vi "Digital chip test.vi"() -> ()   [LabVIEW 2019]
uses:
  <vilib>/VirtualBench/VirtualBench.lvlib
  <vilib>/Utility/error.llb/DialogType.ctl
  <vilib>/VirtualBench/_PS Configure Voltage Output0.vi
  <vilib>/VirtualBench/_DMM Configure Measurement2.vi
  <vilib>/VirtualBench/_MSO Configure Analog Channel28.vi
  <vilib>/VirtualBench/_FGEN Configure Standard Waveform4.vi
  <vilib>/VirtualBench/_MSO Configure Timing12.vi
  <vilib>/DigilentWF/DigilentWF.lvlib
panel:
  out "VOL(V)":dbl format="%#.2f"
  in  "图表选项卡":enum32{"VOH", "VOL", "电压传输特性"}(tab)
  out "VOH":string[][](table)=[["0", "0", "0", "0"]]
  out "VOL(V)":string[][](table)=[["0", "0", "0", "0"]]
  out "波形图":waveform(dbl)[](graph)
  out "VOH(V)":dbl format="%#.2f"
  out "IIH(μA)":dbl format="%#.2f"
  out "IIL(mA)":dbl format="%#.2f"
  out "ICCH(mA)":dbl format="%#.2f"
  in  "测试参数选项卡":T1(tab)=enum."VOL"
  in  "通道一电压":T2
  in  "测量模式":T3(ring)=enum."DC Current"
  in  "通道一电压 2":T2
  in  "测量模式":T3(ring)=enum."DC Current"
  in  "通道一电压":T2
  in  "测量模式":T3(ring)=enum."DC Current"
  in  "通道一电压 2":T4
  in  "通道一电压":T2
  in  "测量模式":T3(ring)=enum."DC Current"
  in  "通道一电压2":T4
  in  "通道一电压 4":T2
  in  "测量模式":T3(ring)=enum."DC Current"
  in  "通道一电压2 2":T4
  in  "测量模式":T3(ring)=enum."DC Current"
  in  "通道一电压2":T4
  in  "通道一电压":T2
  in  "通道一电压1":T2
  in  "通道一电压2 4":T4
  in  "Amplitude":dbl caption="Amplitude (no change)"
  in  "DC Offset":dbl caption="DC Offset (no change)"
  in  "测量范围":dbl caption="Vertical Range (no change)"
  in  "示波器通道选择":tag caption="Channel"
  in  "Waveform Function":i32(ring) caption="Waveform Function (no change)" items=["Sine", "Square", "Triangle/Ramp", "DC"]
  in  "Frequency":dbl caption="Frequency (no change)"
  out "ICCL(mA)":dbl format="%#.2f"
  in  "测试机台选择":tag="VB8012-3115AD9"
  in  "开始测试":bool caption="Start"
  out "测试进度":u8(slide)=100 caption="Testing..." scale=0.0..100.0
  # "基于IECUBE-3839的74芯片自动化测试程序"
  # "硬件配置"
  # "DUT测试参数"
  # "任务点\n1\n配\n置\n仪\n器\n参\n数"
  # "电源配置"
  # "数字万用表配置"
  # "电源配置"
  # "数字万用表配置"
  # "电源配置"
  # "数字万用表配置"
  # "电源配置"
  # "数字万用表配置"
  # "电源配置"
  # "数字万用表配置"
  # "电源配置"
  # "数字万用表配置"
  # "电源配置"
  # "信号源配置"
  # "示波器配置"
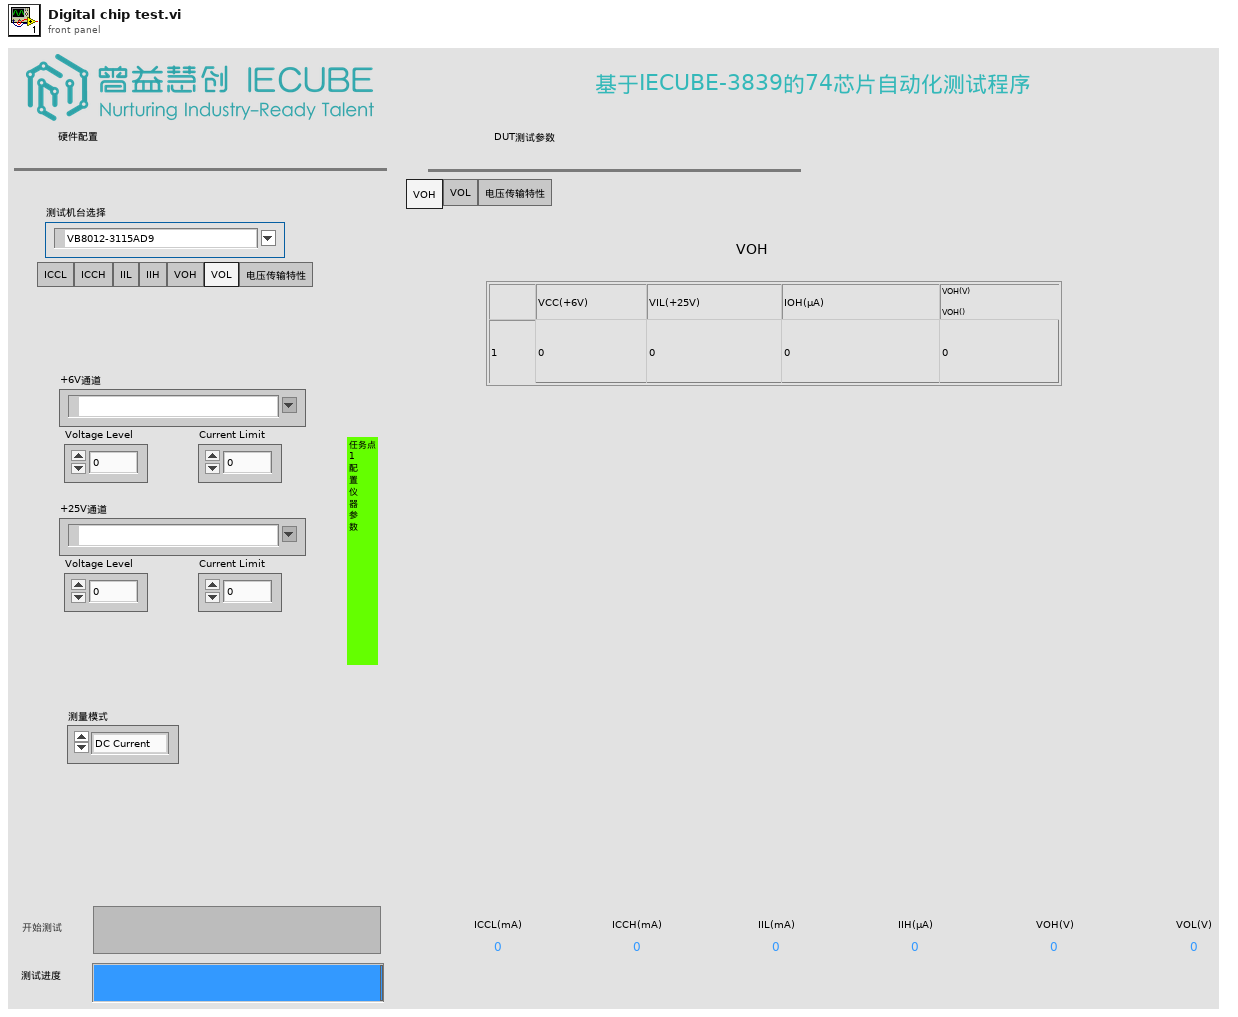
[diagram p1: front panel]
types:
  T1 = enum32{"ICCL", "ICCH", "IIL", "IIH", "VOH", "VOL", "电压传输特性"}
  T2 = cluster{"+6V通道":tag, "Voltage Level":dbl, "Current Limit":dbl}
  T3 = enum16{"DC Volts", "AC Volts", "DC Current", "AC Current", "Resistance", "Diode"}
  T4 = cluster{"+25V通道":tag, "Voltage Level":dbl, "Current Limit":dbl}
  T5 = enum16{"ICCL", "ICCH", "IIL", "IIH", "VOH", "VOL", "电压传输特性"}
  T6 = typedef "DialogType.ctl" = u16
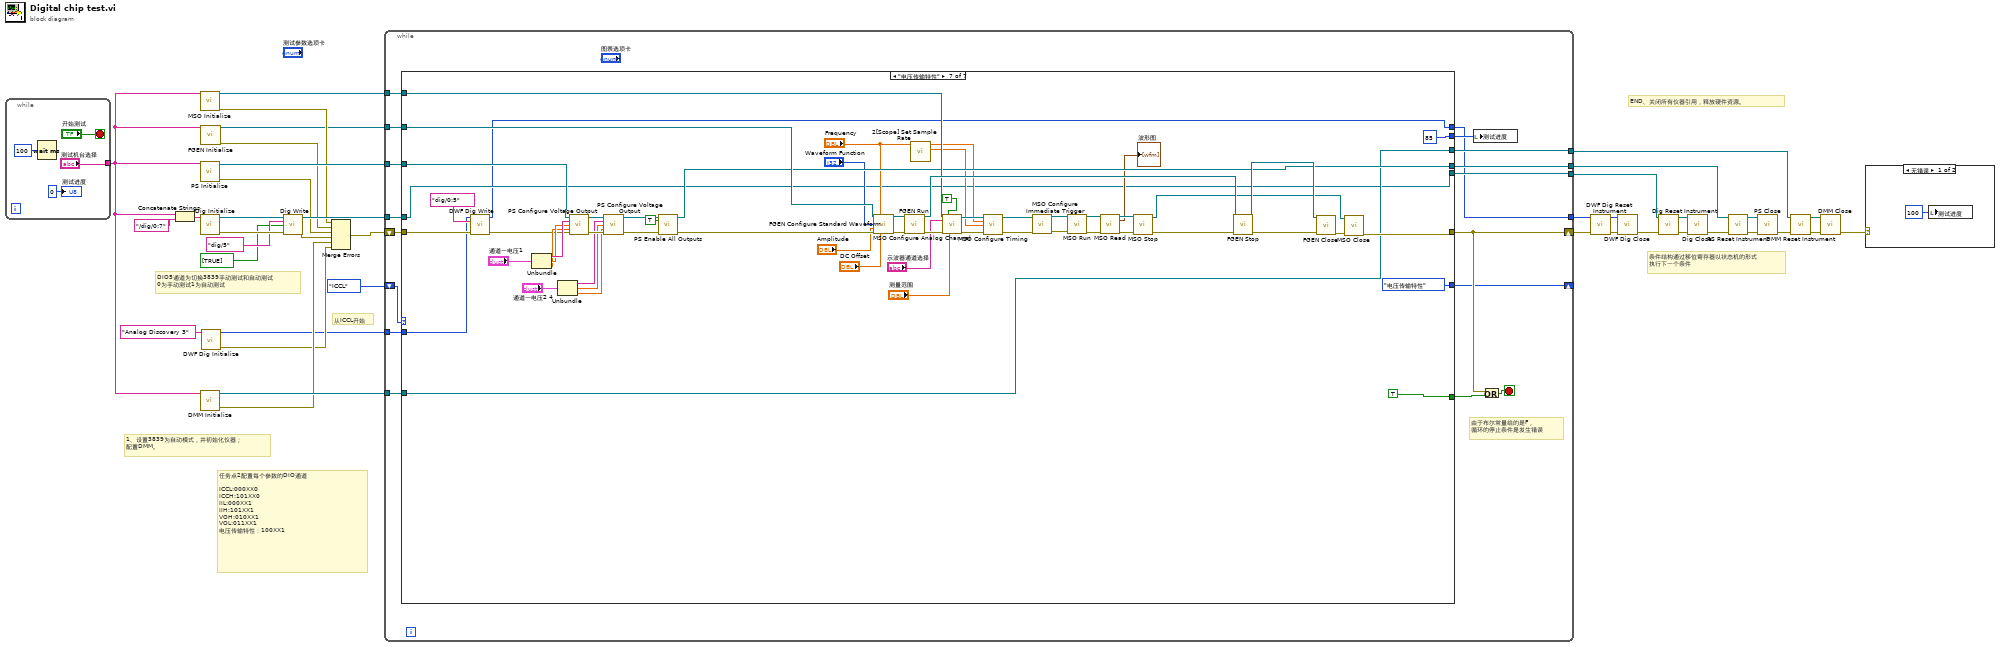
[diagram p0: block diagram]
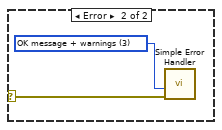
[diagram p2: hidden frame]
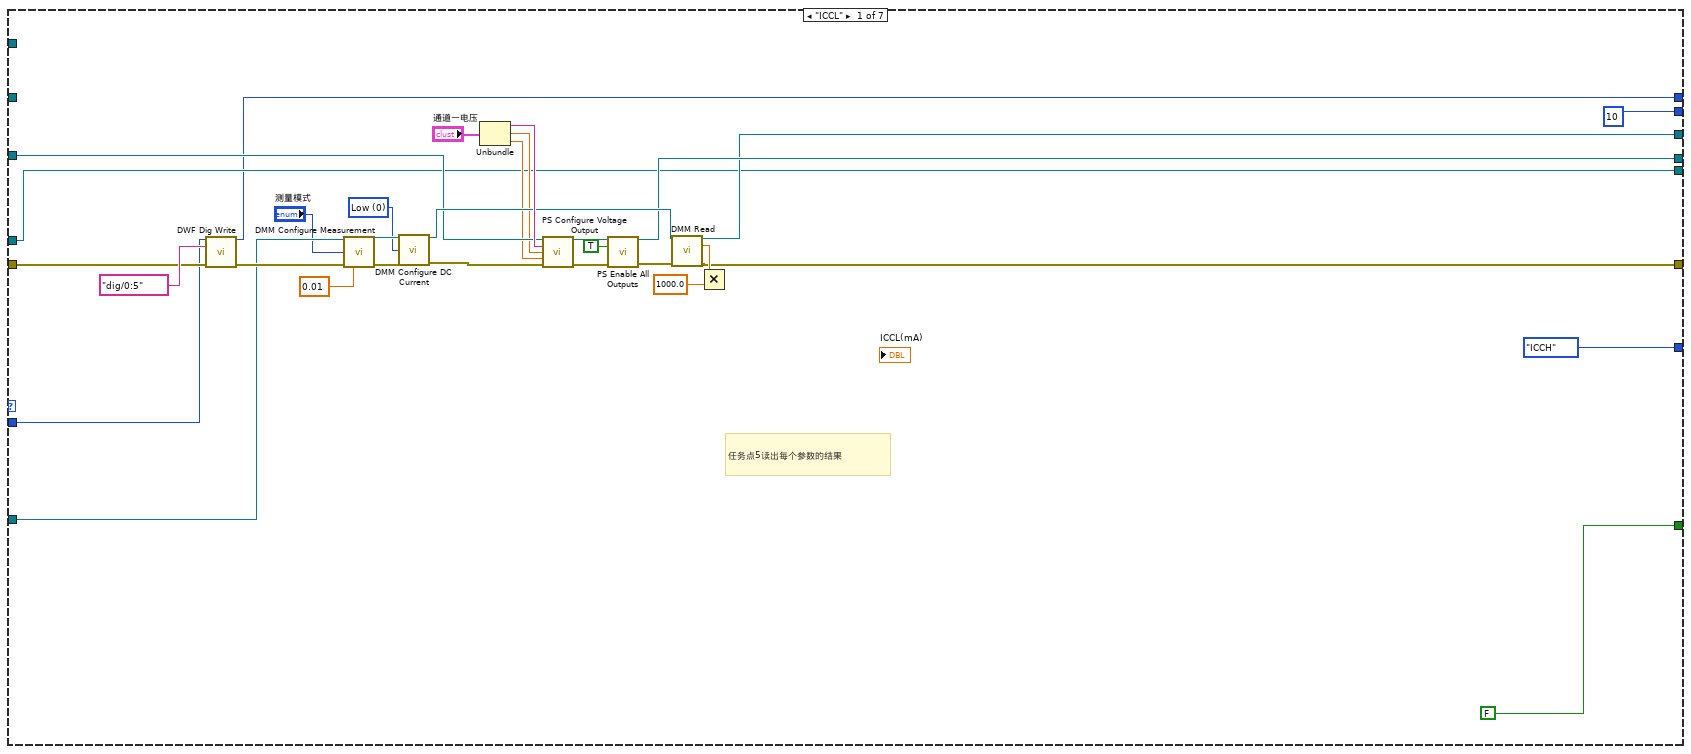
[diagram p3: hidden frame]
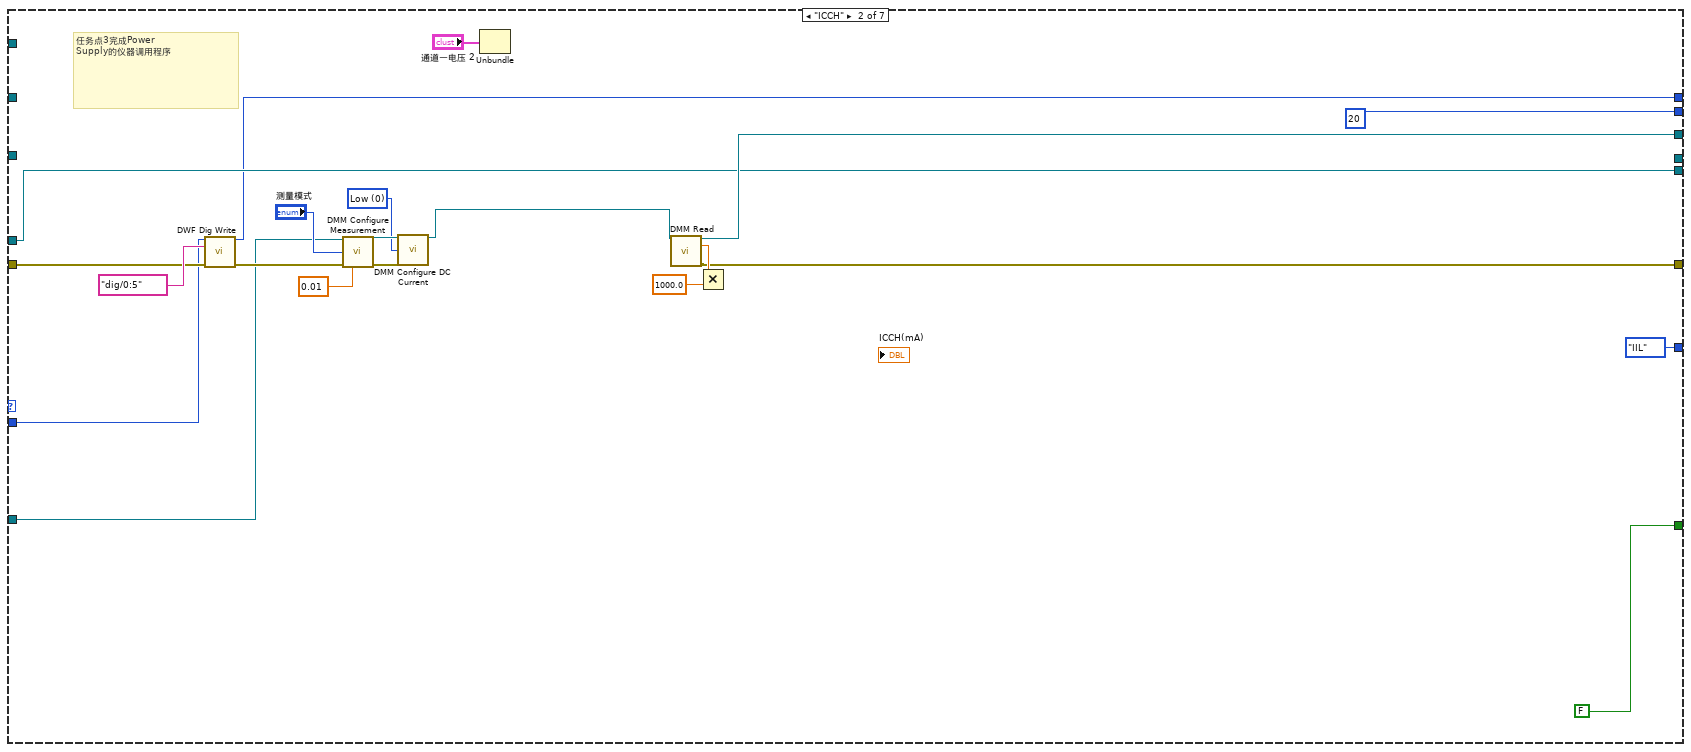
[diagram p4: hidden frame]
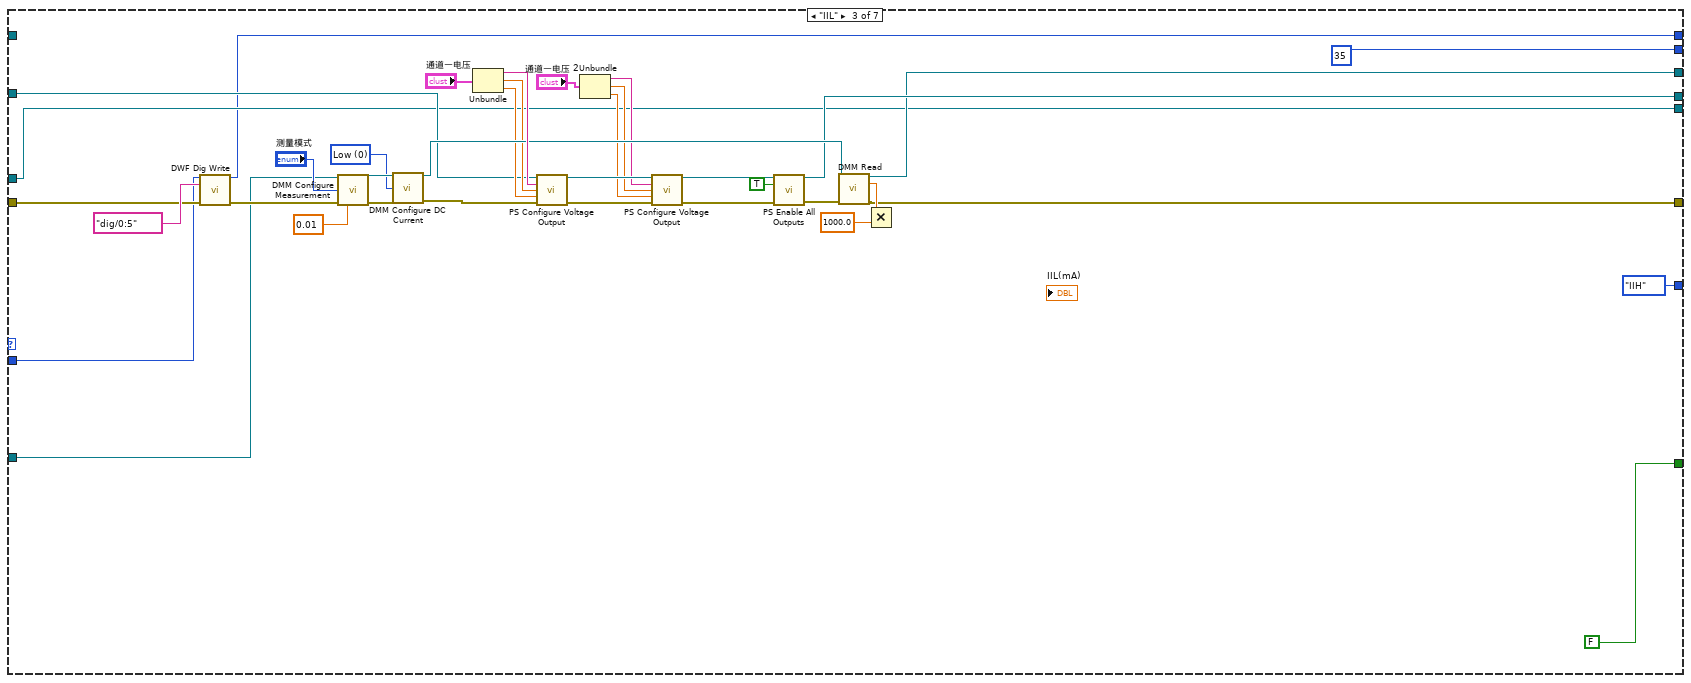
[diagram p5: hidden frame]
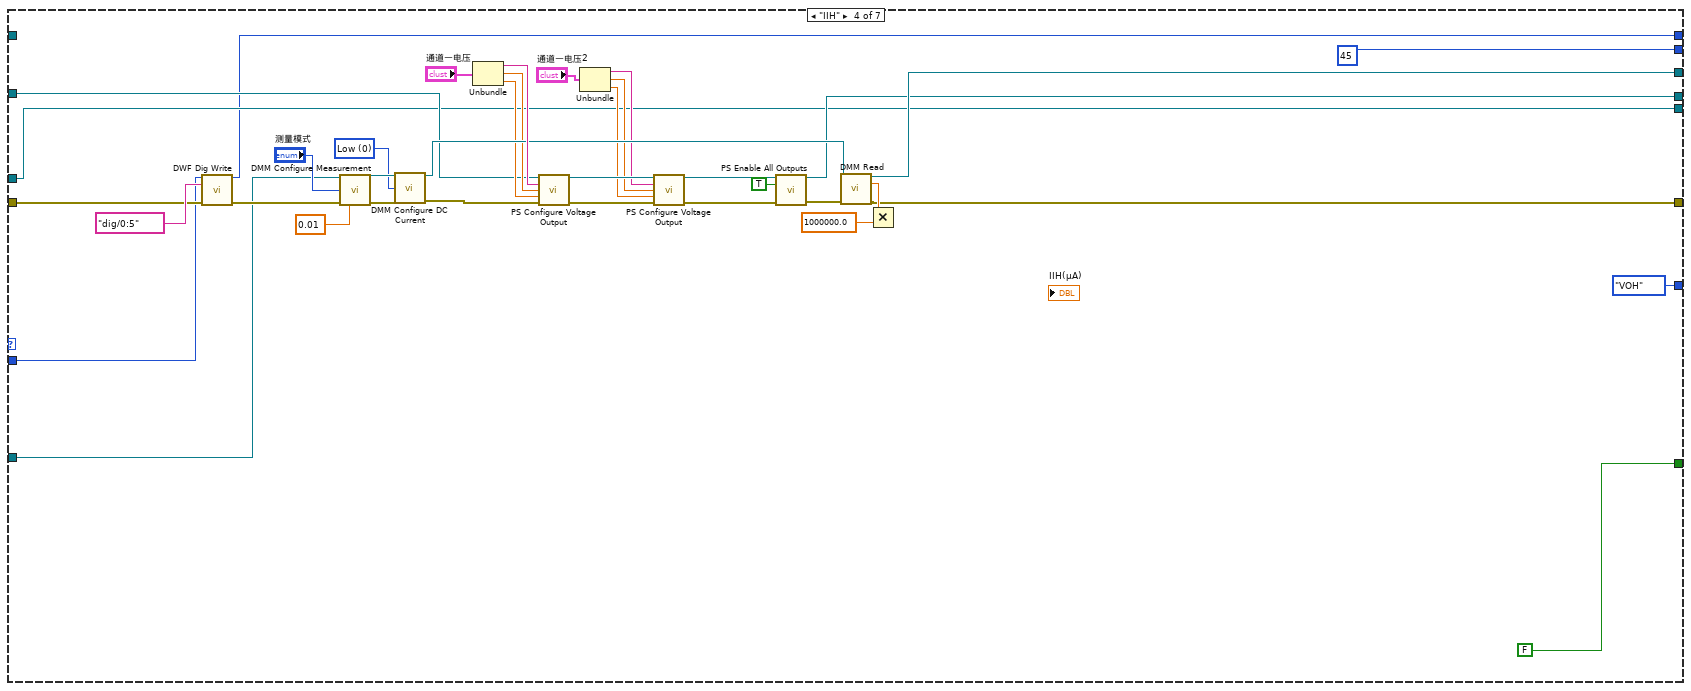
[diagram p6: hidden frame]
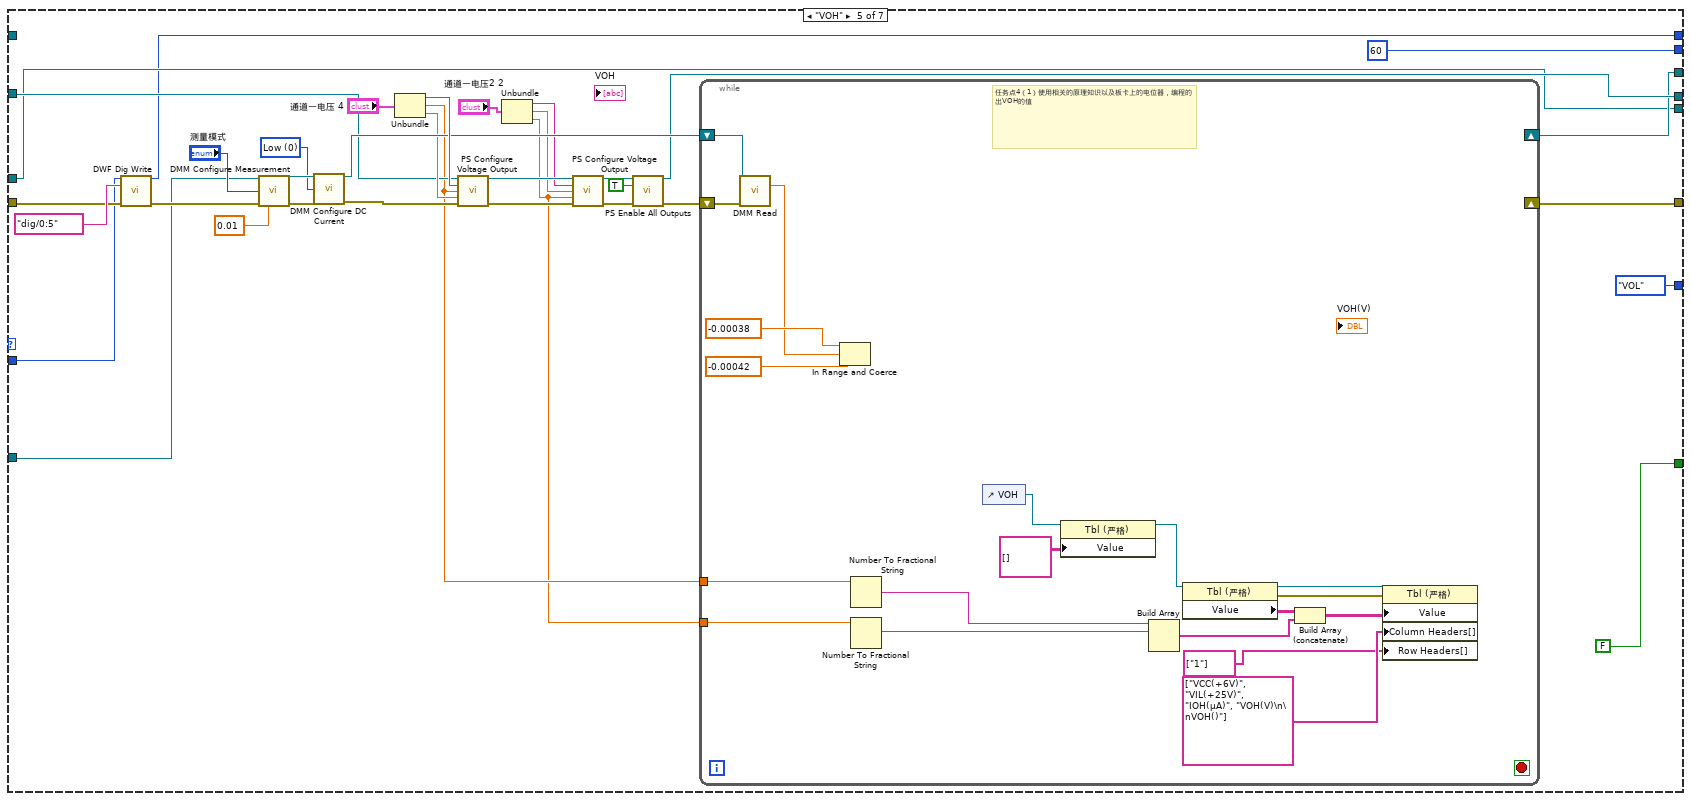
[diagram p7: hidden frame]
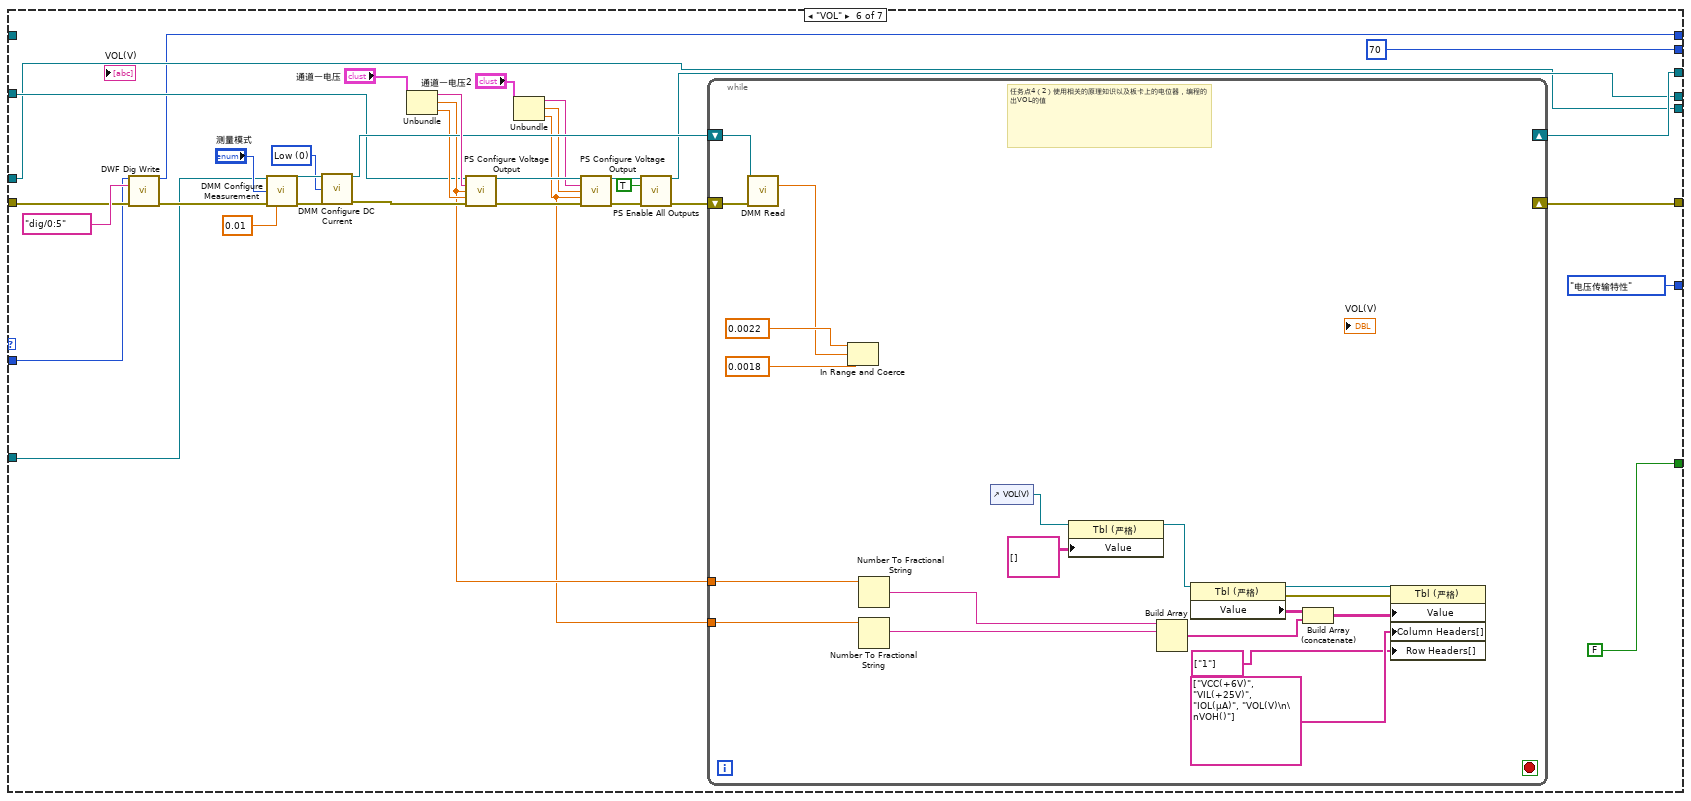
[diagram p8: hidden frame]
diagram:
  # "任务点2配置每个参数的DIO通道\n\nICCL:000XX0\nICCH:101XX0\nIIL:000XX1\nIIH:101XX1\nVOH:010XX1\nVOL:011XX1\n电压传输特性：100XX1"
  # "条件结构通过移位寄存器以状态机的形式\n执行下一个条件"
  # "从ICCL开始"
  # "DIO5通道为切换3839手动测试和自动测试\n0为手动测试1为自动测试"
  # "END、关闭所有仪器引用，释放硬件资源。"
  # "1、设置3839为自动模式，并初始化仪器；\n配置DMM。"
  n1 = while {
    tunnel: ["测试机台选择"] -> w14
    stop <- "开始测试" stop-if-true
    n2 = Wait (ms)(milliseconds to wait=u32 100 ("等待时间（毫秒）")) -> ()  [unwired: 1 out]
    "测试进度" <- u8 0 ("测试进度")
  }
  n3 = Concatenate Strings(w14, "/dig/0:7" ("字符串")) -> (w34:string)
  n4 = call <vilib>:"MSO Initialize.vi"("Device Name"=w14) -> ("Instrument Handle Out"=w11:refnum<k21>, "Error Out"=w12:errorcluster)  [unwired: 13 in]
  n5 = call <vilib>:"PS Initialize.vi"("Device Name"=w14) -> ("Instrument Handle Out"=w33:refnum<k21>, "Error Out"=w30:errorcluster)  [unwired: 13 in]
  n6 = call <vilib>:"Dig Initialize.vi"("Lines"=w34) -> ("Instrument Handle Out"=w39:refnum<k21>, "Error Out"=w38:errorcluster)  [unwired: 13 in]
  n7 = call <vilib>:"DMM Initialize.vi"("Device Name"=w14) -> ("Instrument Handle Out"=w28:refnum<k21>, "Error Out"=w27:errorcluster)  [unwired: 13 in]
  n8 = call <vilib>:"FGEN Initialize.vi"("Device Name"=w14) -> ("Instrument Handle Out"=w10:refnum<k21>, "Error Out"=w13:errorcluster)  [unwired: 13 in]
  n9 = call <vilib>:"DWF Dig Initialize.vi"("Device Name/Lines"="Analog Discovery 3") -> ("Instrument Handle Out"=w6:u32, "Error Out"=w7:errorcluster)  [unwired: 13 in]
  n10 = call <vilib>:"Dig Write.vi"("Instrument Handle In"=w39, "Lines"=tag "dig/5", "Data"=bool[] [TRUE], "Error In"=w38) -> ("Instrument Handle Out"=w32:refnum<k21>, "Error Out"=w29:errorcluster)  [unwired: 10 in]
  n11 = Merge Errors(w12, w13, w30, w29, w27, w7) -> (w31:errorcluster)
  n12 = while {
    tunnel: w32 -> [w44]
    tunnel: w33 -> [w58]
    tunnel: w28 -> [w60]
    shift-right: [w52] -> w5
    shift-left: w31 -> [w59]
    tunnel: [w51] -> w17
    tunnel: [w57] -> w23
    tunnel: [w53] -> w15
    tunnel: w11 -> [w50]
    tunnel: w10 -> [w49]
    shift-right: [w47] -> _
    shift-left: T5."ICCL" -> [w48]
    tunnel: w6 -> [w46]
    tunnel: [w45] -> w1
    stop <- w54 stop-if-true
    # "由于布尔常量给的是F，\n循环的停止条件是发生错误"
    n13 = case shown="\"电压传输特性\"" w48 {
      tunnel: w60 -> [w75 w100 w132 w161 w200 w262 w329]
      tunnel: w59 -> [w77 w101 w133 w162 w201 w263 w340]
      tunnel: w44 -> [w63 w94 w117 w154 w191 w253 w316]
      tunnel: w58 -> [w73 _ w134 w163 w202 w264 w338]
      tunnel: [w65 w99 w129 w159 w197 w260 w329] -> w51
      tunnel: [w72 _ w130 w158 w198 w259 w332] -> w57
      tunnel: [u8 10 ("测试进度") u8 20 ("测试进度") u8 35 ("测试进度") u8 45 ("测试进度") u8 60 ("测试进度") u8 70 ("测试进度") u8 85 ("测试进度")] -> w56
      tunnel: [FALSE FALSE FALSE FALSE FALSE FALSE TRUE] -> w55
      tunnel: [w63 w94 w117 w154 w191 w253 w316] -> w53
      tunnel: [w66 w97 w131 w157 w199 w261 w330] -> w52
      tunnel: w50 -> [_ _ _ _ _ _ w335]
      tunnel: w49 -> [_ _ _ _ _ _ w334]
      tunnel: [T5."ICCH" T5."IIL" T5."IIH" T5."VOH" T5."VOL" T5."电压传输特性" T5."电压传输特性"] -> w47
      tunnel: w46 -> [w61 w92 w116 w153 w190 w252 w315]
      tunnel: [w62 w93 w115 w152 w189 w251 w314] -> w45
      frame "ICCL" {
        w88 = 0 items=["Low", "High"] ("Auto Range Terminal")
        # "任务点5读出每个参数的结果"
        n14 = call <vilib>:"DWF Dig Write.vi"("Instrument Handle In"=w61, "Lines"=tag "dig/0:5", "Error In"=w77) -> ("Instrument Handle Out"=w62:u32, "Error Out"=w76:errorcluster)  [unwired: 11 in]
        n15 = call-poly <vilib>:"DMM Configure Measurement.vi"("Instrument Handle In"=w75, "Function"="测量模式", "Error In"=w76, "Manual Range"=0.01) -> ("Instrument Handle Out"=w89:refnum<k21>, "Error Out"=w90:errorcluster)  [unwired: 10 in]
        n16 = call <vilib>:"DMM Configure DC Current.vi"("Instrument Handle In"=w89, "Auto Range Terminal"=w88, "Error In"=w90) -> ("Instrument Handle Out"=w81:refnum<k21>, "Error Out"=w74:errorcluster)  [unwired: 11 in]
        n17 = Unbundle("通道一电压") -> ("+6V通道"=w85:tag, "Voltage Level"=w68:dbl, "Current Limit"=w69:dbl)
        n18 = call-poly <vilib>:"PS Configure Voltage Output.vi"("Instrument Handle In"=w73, "Channel"=w85, "Voltage Level"=w68, "Current Limit"=w69, "Error In"=w74) -> ("Instrument Handle Out"=w84:refnum<k21>, "Error Out"=w83:errorcluster)  [unwired: 9 in]
        n19 = call <vilib>:"PS Enable All Outputs.vi"("Instrument Handle In"=w84, "Enable Outputs"=TRUE, "Error In"=w83) -> ("Instrument Handle Out"=w72:refnum<k21>, "Error Out"=w80:errorcluster)  [unwired: 11 in]
        n20 = call <vilib>:"DMM Read.vi"("Instrument Handle In"=w81, "Error In"=w80) -> ("Instrument Handle Out"=w65:refnum<k21>, "Measurement"=w79:dbl, "Error Out"=w66:errorcluster)  [unwired: 11 in]
        n21 = Multiply(x=w79, y=1000.0) -> ()  [unwired: 1 out]
      }
      frame "ICCH" {
        w112 = 0 items=["Low", "High"] ("Auto Range Terminal")
        # "任务点3完成Power Supply的仪器调用程序"
        n22 = call <vilib>:"DWF Dig Write.vi"("Instrument Handle In"=w92, "Lines"=tag "dig/0:5", "Error In"=w101) -> ("Instrument Handle Out"=w93:u32, "Error Out"=w105:errorcluster)  [unwired: 11 in]
        n23 = call-poly <vilib>:"DMM Configure Measurement.vi"("Instrument Handle In"=w100, "Function"="测量模式", "Error In"=w105, "Manual Range"=0.01) -> ("Instrument Handle Out"=w113:refnum<k21>, "Error Out"=w114:errorcluster)  [unwired: 10 in]
        n24 = call <vilib>:"DMM Configure DC Current.vi"("Instrument Handle In"=w113, "Auto Range Terminal"=w112, "Error In"=w114) -> ("Instrument Handle Out"=w109:refnum<k21>, "Error Out"=w104:errorcluster)  [unwired: 11 in]
        n25 = Unbundle("通道一电压 2") -> ()  [unwired: 3 out]
        n26 = call <vilib>:"DMM Read.vi"("Instrument Handle In"=w109) -> ("Instrument Handle Out"=w99:refnum<k21>, "Measurement"=w107:dbl, "Error In"=w108:errorcluster, "Error Out"=w97:errorcluster)  [unwired: 11 in]
        n27 = Multiply(x=w107, y=1000.0) -> ()  [unwired: 1 out]
      }
      frame "IIL" {
        w149 = 0 items=["Low", "High"] ("Auto Range Terminal")
        n28 = call <vilib>:"DWF Dig Write.vi"("Instrument Handle In"=w116, "Lines"=tag "dig/0:5", "Error In"=w133) -> ("Instrument Handle Out"=w115:u32, "Error Out"=w140:errorcluster)  [unwired: 11 in]
        n29 = call-poly <vilib>:"DMM Configure Measurement.vi"("Instrument Handle In"=w132, "Function"="测量模式", "Error In"=w140, "Manual Range"=0.01) -> ("Instrument Handle Out"=w150:refnum<k21>, "Error Out"=w151:errorcluster)  [unwired: 10 in]
        n30 = call <vilib>:"DMM Configure DC Current.vi"("Instrument Handle In"=w150, "Auto Range Terminal"=w149, "Error In"=w151) -> ("Instrument Handle Out"=w144:refnum<k21>, "Error Out"=w139:errorcluster)  [unwired: 11 in]
        n31 = Unbundle("通道一电压") -> ("+6V通道"=w146:tag, "Voltage Level"=w136:dbl, "Current Limit"=w137:dbl)
        n32 = call-poly <vilib>:"PS Configure Voltage Output.vi"("Instrument Handle In"=w134, "Channel"=w146, "Voltage Level"=w136, "Current Limit"=w137, "Error In"=w139) -> ("Instrument Handle Out"=w126:refnum<k21>, "Error Out"=w123:errorcluster)  [unwired: 9 in]
        n33 = Unbundle("通道一电压 2") -> ("+25V通道"=w122:tag, "Voltage Level"=w121:dbl, "Current Limit"=w120:dbl)
        n34 = call-poly <vilib>:"PS Configure Voltage Output.vi"("Instrument Handle In"=w126, "Channel"=w122, "Voltage Level"=w121, "Current Limit"=w120, "Error In"=w123) -> ("Instrument Handle Out"=w125:refnum<k21>, "Error Out"=w124:errorcluster)  [unwired: 9 in]
        n35 = call <vilib>:"PS Enable All Outputs.vi"("Instrument Handle In"=w125, "Enable Outputs"=TRUE, "Error In"=w124) -> ("Instrument Handle Out"=w130:refnum<k21>, "Error Out"=w143:errorcluster)  [unwired: 11 in]
        n36 = call <vilib>:"DMM Read.vi"("Instrument Handle In"=w144, "Error In"=w143) -> ("Instrument Handle Out"=w129:refnum<k21>, "Measurement"=w142:dbl, "Error Out"=w131:errorcluster)  [unwired: 11 in]
        n37 = Multiply(x=w142, y=1000.0) -> ()  [unwired: 1 out]
      }
      frame "IIH" {
        w186 = 0 items=["Low", "High"] ("Auto Range Terminal")
        n38 = call <vilib>:"DWF Dig Write.vi"("Instrument Handle In"=w153, "Lines"=tag "dig/0:5", "Error In"=w162) -> ("Instrument Handle Out"=w152:u32, "Error Out"=w177:errorcluster)  [unwired: 11 in]
        n39 = call-poly <vilib>:"DMM Configure Measurement.vi"("Instrument Handle In"=w161, "Function"="测量模式", "Error In"=w177, "Manual Range"=0.01) -> ("Instrument Handle Out"=w187:refnum<k21>, "Error Out"=w188:errorcluster)  [unwired: 10 in]
        n40 = call <vilib>:"DMM Configure DC Current.vi"("Instrument Handle In"=w187, "Auto Range Terminal"=w186, "Error In"=w188) -> ("Instrument Handle Out"=w181:refnum<k21>, "Error Out"=w176:errorcluster)  [unwired: 11 in]
        n41 = Unbundle("通道一电压") -> ("+6V通道"=w183:tag, "Voltage Level"=w173:dbl, "Current Limit"=w174:dbl)
        n42 = call-poly <vilib>:"PS Configure Voltage Output.vi"("Instrument Handle In"=w163, "Channel"=w183, "Voltage Level"=w173, "Current Limit"=w174, "Error In"=w176) -> ("Instrument Handle Out"=w170:refnum<k21>, "Error Out"=w167:errorcluster)  [unwired: 9 in]
        n43 = Unbundle("通道一电压2") -> ("+25V通道"=w166:tag, "Voltage Level"=w165:dbl, "Current Limit"=w164:dbl)
        n44 = call-poly <vilib>:"PS Configure Voltage Output.vi"("Instrument Handle In"=w170, "Channel"=w166, "Voltage Level"=w165, "Current Limit"=w164, "Error In"=w167) -> ("Instrument Handle Out"=w169:refnum<k21>, "Error Out"=w168:errorcluster)  [unwired: 9 in]
        n45 = call <vilib>:"PS Enable All Outputs.vi"("Instrument Handle In"=w169, "Enable Outputs"=TRUE, "Error In"=w168) -> ("Instrument Handle Out"=w158:refnum<k21>, "Error Out"=w180:errorcluster)  [unwired: 11 in]
        n46 = call <vilib>:"DMM Read.vi"("Instrument Handle In"=w181, "Error In"=w180) -> ("Instrument Handle Out"=w159:refnum<k21>, "Measurement"=w179:dbl, "Error Out"=w157:errorcluster)  [unwired: 11 in]
        n47 = Multiply(x=w179, y=1000000.0) -> ()  [unwired: 1 out]
      }
      frame "VOH" {
        w221 = 0 items=["Low", "High"] ("Auto Range Terminal")
        n48 = call <vilib>:"DWF Dig Write.vi"("Instrument Handle In"=w190, "Lines"=tag "dig/0:5", "Error In"=w201) -> ("Instrument Handle Out"=w189:u32, "Error Out"=w214:errorcluster)  [unwired: 11 in]
        n49 = call-poly <vilib>:"DMM Configure Measurement.vi"("Instrument Handle In"=w200, "Function"="测量模式", "Error In"=w214, "Manual Range"=0.01) -> ("Instrument Handle Out"=w222:refnum<k21>, "Error Out"=w223:errorcluster)  [unwired: 10 in]
        n50 = call <vilib>:"DMM Configure DC Current.vi"("Instrument Handle In"=w222, "Auto Range Terminal"=w221, "Error In"=w223) -> ("Instrument Handle Out"=w216:refnum<k21>, "Error Out"=w213:errorcluster)  [unwired: 11 in]
        n51 = Unbundle("通道一电压 4") -> ("+6V通道"=w218:tag, "Voltage Level"=w195:dbl, "Current Limit"=w211:dbl)
        n52 = call-poly <vilib>:"PS Configure Voltage Output.vi"("Instrument Handle In"=w202, "Channel"=w218, "Voltage Level"=w195, "Current Limit"=w211, "Error In"=w213) -> ("Instrument Handle Out"=w208:refnum<k21>, "Error Out"=w205:errorcluster)  [unwired: 9 in]
        n53 = Unbundle("通道一电压2 2") -> ("+25V通道"=w204:tag, "Voltage Level"=w203:dbl, "Current Limit"=w194:dbl)
        n54 = call-poly <vilib>:"PS Configure Voltage Output.vi"("Instrument Handle In"=w208, "Channel"=w204, "Voltage Level"=w203, "Current Limit"=w194, "Error In"=w205) -> ("Instrument Handle Out"=w207:refnum<k21>, "Error Out"=w206:errorcluster)  [unwired: 9 in]
        n55 = call <vilib>:"PS Enable All Outputs.vi"("Instrument Handle In"=w207, "Enable Outputs"=TRUE, "Error In"=w206) -> ("Instrument Handle Out"=w198:refnum<k21>, "Error Out"=w215:errorcluster)  [unwired: 11 in]
        n56 = while {
          shift-right: [w243] -> w197
          shift-left: w216 -> [w250]
          shift-right: [w242] -> w199
          shift-left: w215 -> [w249]
          tunnel: w195 -> [w226]
          tunnel: w194 -> [w225]
          stop <- w224 stop-if-true
          # "任务点4（1）使用相关的原理知识以及板卡上的电位器，编程的出VOH的值"
          n57 = call <vilib>:"DMM Read.vi"("Instrument Handle In"=w250, "Error In"=w249) -> ("Instrument Handle Out"=w245:refnum<k21>, "Measurement"=w241:dbl, "Error Out"=w244:errorcluster)  [unwired: 11 in]
          n58 = In Range and Coerce(upper limit=-0.00038 ("上限"), x=w241, lower limit=-0.00042 ("下限")) -> (In Range?=w246:bool)  [unwired: 1 out]
          n59 = Number To Fractional String(number=w226) -> (F-format string=w240:string)  [unwired: 3 in]
          n60 = Number To Fractional String(number=w225) -> (F-format string=w233:string)  [unwired: 3 in]
          n61 = control-ref of="VOH"() -> (w229:refnum<vi>)
          n62 = property class="Tbl (严格)"(reference=w229, "Value"=string[][] [] ("值")) -> (reference out=w235:refnum<vi>)  [unwired: 1 in, 1 out]
          n63 = Build Array(w240, w233) -> (w234:string[], w227:string, w228:string)
          n64 = property class="Tbl (严格)"(reference=w235) -> (reference out=w238:refnum<vi>, error out=w239:errorcluster, "Value"=w237:string[][])  [unwired: 1 in]
          n65 = Build Array (concatenate)(w237, w234) -> (w236:string[][])
          n66 = property class="Tbl (严格)"(reference=w238, error in=w239, "Value"=w236, "Column Headers[]"=string[] ["VCC(+6V)", "VIL(+25V)", "IOH(μA)", "VOH(V)\n\nVOH()"] ("列首字符串[]"), "Row Headers[]"=string[] ["1"] ("列首字符串[]")) -> ()  [unwired: 2 out]
        }
      }
      frame "VOL" {
        w283 = 0 items=["Low", "High"] ("Auto Range Terminal")
        n67 = call <vilib>:"DWF Dig Write.vi"("Instrument Handle In"=w252, "Lines"=tag "dig/0:5", "Error In"=w263) -> ("Instrument Handle Out"=w251:u32, "Error Out"=w276:errorcluster)  [unwired: 11 in]
        n68 = call-poly <vilib>:"DMM Configure Measurement.vi"("Instrument Handle In"=w262, "Function"="测量模式", "Error In"=w276, "Manual Range"=0.01) -> ("Instrument Handle Out"=w284:refnum<k21>, "Error Out"=w285:errorcluster)  [unwired: 10 in]
        n69 = call <vilib>:"DMM Configure DC Current.vi"("Instrument Handle In"=w284, "Auto Range Terminal"=w283, "Error In"=w285) -> ("Instrument Handle Out"=w278:refnum<k21>, "Error Out"=w275:errorcluster)  [unwired: 11 in]
        n70 = Unbundle("通道一电压") -> ("+6V通道"=w280:tag, "Voltage Level"=w266:dbl, "Current Limit"=w273:dbl)
        n71 = call-poly <vilib>:"PS Configure Voltage Output.vi"("Instrument Handle In"=w264, "Channel"=w280, "Voltage Level"=w266, "Current Limit"=w273, "Error In"=w275) -> ("Instrument Handle Out"=w272:refnum<k21>, "Error Out"=w269:errorcluster)  [unwired: 9 in]
        n72 = Unbundle("通道一电压2") -> ("+25V通道"=w268:tag, "Voltage Level"=w267:dbl, "Current Limit"=w265:dbl)
        n73 = call-poly <vilib>:"PS Configure Voltage Output.vi"("Instrument Handle In"=w272, "Channel"=w268, "Voltage Level"=w267, "Current Limit"=w265, "Error In"=w269) -> ("Instrument Handle Out"=w271:refnum<k21>, "Error Out"=w270:errorcluster)  [unwired: 9 in]
        n74 = call <vilib>:"PS Enable All Outputs.vi"("Instrument Handle In"=w271, "Enable Outputs"=TRUE, "Error In"=w270) -> ("Instrument Handle Out"=w259:refnum<k21>, "Error Out"=w277:errorcluster)  [unwired: 11 in]
        n75 = while {
          shift-right: [w306] -> w260
          shift-left: w278 -> [w313]
          shift-right: [w305] -> w261
          shift-left: w277 -> [w312]
          tunnel: w266 -> [w289]
          tunnel: w265 -> [w288]
          stop <- w286 stop-if-true
          # "任务点4（2）使用相关的原理知识以及板卡上的电位器，编程的出VOL的值"
          n76 = call <vilib>:"DMM Read.vi"("Instrument Handle In"=w313, "Error In"=w312) -> ("Instrument Handle Out"=w308:refnum<k21>, "Measurement"=w304:dbl, "Error Out"=w307:errorcluster)  [unwired: 11 in]
          n77 = In Range and Coerce(upper limit=0.0022 ("上限"), x=w304, lower limit=0.0018 ("下限")) -> (In Range?=w309:bool)  [unwired: 1 out]
          n78 = Number To Fractional String(number=w289) -> (F-format string=w303:string)  [unwired: 3 in]
          n79 = Number To Fractional String(number=w288) -> (F-format string=w296:string)  [unwired: 3 in]
          n80 = control-ref of="VOL(V)"() -> (w292:refnum<vi>)
          n81 = property class="Tbl (严格)"(reference=w292, "Value"=string[][] [] ("值")) -> (reference out=w298:refnum<vi>)  [unwired: 1 in, 1 out]
          n82 = Build Array(w303, w296) -> (w297:string[], w290:string, w291:string)
          n83 = property class="Tbl (严格)"(reference=w298) -> (reference out=w301:refnum<vi>, error out=w302:errorcluster, "Value"=w300:string[][])  [unwired: 1 in]
          n84 = Build Array (concatenate)(w300, w297) -> (w299:string[][])
          n85 = property class="Tbl (严格)"(reference=w301, error in=w302, "Value"=w299, "Column Headers[]"=string[] ["VCC(+6V)", "VIL(+25V)", "IOL(μA)", "VOL(V)\n\nVOH()"] ("列首字符串[]"), "Row Headers[]"=string[] ["1"] ("列首字符串[]")) -> ()  [unwired: 2 out]
        }
      }
      frame "电压传输特性" {
        n86 = call <vilib>:"DWF Dig Write.vi"("Instrument Handle In"=w315, "Lines"=tag "dig/0:5", "Error In"=w340) -> ("Instrument Handle Out"=w314:u32, "Error Out"=w333:errorcluster)  [unwired: 11 in]
        n87 = Unbundle("通道一电压1") -> ("+6V通道"=w369:tag, "Voltage Level"=w368:dbl, "Current Limit"=w367:dbl)
        n88 = Unbundle("通道一电压2 4") -> ("+25V通道"=w345:tag, "Voltage Level"=w344:dbl, "Current Limit"=w343:dbl)
        n89 = call-poly <vilib>:"PS Configure Voltage Output.vi"("Instrument Handle In"=w338, "Channel"=w369, "Voltage Level"=w368, "Current Limit"=w367, "Error In"=w333) -> ("Instrument Handle Out"=w363:refnum<k21>, "Error Out"=w364:errorcluster)  [unwired: 9 in]
        n90 = call-poly <vilib>:"PS Configure Voltage Output.vi"("Instrument Handle In"=w363, "Channel"=w345, "Voltage Level"=w344, "Current Limit"=w343) -> ("Instrument Handle Out"=w346:refnum<k21>)  [unwired: 10 in, 1 out]
        n91 = call <vilib>:"PS Enable All Outputs.vi"("Instrument Handle In"=w346, "Enable Outputs"=TRUE, "Error In"=w364) -> ("Instrument Handle Out"=w332:refnum<k21>, "Error Out"=w342:errorcluster)  [unwired: 11 in]
        n92 = call-poly <vilib>:"FGEN Configure Standard Waveform.vi"("Instrument Handle In"=w334, "Frequency"="Frequency", "Waveform Function"="Waveform Function", "Amplitude"="Amplitude", "Error In"=w342, "DC Offset"="DC Offset") -> ("Instrument Handle Out"=w366:refnum<k21>, "Error Out"=w365:errorcluster)  [unwired: 8 in]
        n93 = call <vilib>:"FGEN Run.vi"("Instrument Handle In"=w366, "Error In"=w365) -> ("Instrument Handle Out"=w351:refnum<k21>, "Error Out"=w362:errorcluster)  [unwired: 12 in]
        n94 = call "2[Scope] Set Sample Rate.vi"("Frequency"="Frequency") -> ("Acquistion Time"=w317:dbl, "Sample Rate"=w318:dbl)  [unwired: 9 in]
        n95 = call-poly <vilib>:"MSO Configure Analog Channel.vi"("Instrument Handle In"=w335, "Enable Channel"=TRUE, "Channel"="示波器通道选择", "Error In"=w362, "Vertical Range"="测量范围") -> ("Instrument Handle Out"=w360:refnum<k21>, "Error Out"=w361:errorcluster)  [unwired: 9 in]
        n96 = call-poly <vilib>:"MSO Configure Timing.vi"("Instrument Handle In"=w360, "Sample Rate"=w318, "Acquisition Time (s)"=w317, "Error In"=w361) -> ("Instrument Handle Out"=w359:refnum<k21>, "Error Out"=w358:errorcluster)  [unwired: 10 in]
        n97 = call <vilib>:"MSO Configure Immediate Trigger.vi"("Instrument Handle In"=w359, "Error In"=w358) -> ("Instrument Handle Out"=w357:refnum<k21>, "Error Out"=w356:errorcluster)  [unwired: 12 in]
        n98 = call <vilib>:"MSO Run.vi"("Instrument Handle In"=w357, "Error In"=w356) -> ("Instrument Handle Out"=w354:refnum<k21>, "Error Out"=w355:errorcluster)  [unwired: 12 in]
        n99 = call <vilib>:"MSO Read.vi"("Instrument Handle In"=w354, "Error In"=w355) -> ("Instrument Handle Out"=w353:refnum<k21>, "Analog Waveforms"=→"波形图":waveform(dbl)[], "Error Out"=w352:errorcluster)  [unwired: 8 in, 3 out]
        n100 = call <vilib>:"MSO Stop.vi"("Instrument Handle In"=w353, "Error In"=w352) -> ("Instrument Handle Out"=w348:refnum<k21>, "Error Out"=w341:errorcluster)  [unwired: 12 in]
        n101 = call <vilib>:"FGEN Stop.vi"("Instrument Handle In"=w351, "Error In"=w341) -> ("Instrument Handle Out"=w350:refnum<k21>, "Error Out"=w331:errorcluster)  [unwired: 12 in]
        n102 = call <vilib>:"FGEN Close.vi"("Instrument Handle In"=w350, "Error In"=w331) -> ("Error Out"=w349:errorcluster)  [unwired: 13 in]
        n103 = call <vilib>:"MSO Close.vi"("Instrument Handle In"=w348, "Error In"=w349) -> ("Error Out"=w330:errorcluster)  [unwired: 13 in]
      }
    }
    n104 = local write "测试进度"(w56) -> ()
    n105 = Or(x=w52, y=w55) -> (x .or. y?=w54:bool)
  }
  n106 = call <vilib>:"DWF Dig Reset Instrument.vi"("Instrument Handle In"=w1, "Error In"=w5) -> ("Instrument Handle Out"=w4:u32, "Error Out"=w3:errorcluster)  [unwired: 12 in]
  n107 = call <vilib>:"DWF Dig Close.vi"("Instrument Handle In"=w4, "Error In"=w3) -> ("Error Out"=w2:errorcluster)  [unwired: 13 in]
  n108 = call <vilib>:"Dig Reset Instrument.vi"("Instrument Handle In"=w15, "Error In"=w2) -> ("Instrument Handle Out"=w25:refnum<k21>, "Error Out"=w24:errorcluster)  [unwired: 12 in]
  n109 = call <vilib>:"Dig Close.vi"("Instrument Handle In"=w25, "Error In"=w24) -> ("Error Out"=w22:errorcluster)  [unwired: 13 in]
  n110 = call <vilib>:"PS Reset Instrument.vi"("Instrument Handle In"=w23, "Error In"=w22) -> ("Instrument Handle Out"=w20:refnum<k21>, "Error Out"=w21:errorcluster)  [unwired: 12 in]
  n111 = call <vilib>:"PS Close.vi"("Instrument Handle In"=w20, "Error In"=w21) -> ("Error Out"=w19:errorcluster)  [unwired: 13 in]
  n112 = call <vilib>:"DMM Reset Instrument.vi"("Instrument Handle In"=w17, "Error In"=w19) -> ("Instrument Handle Out"=w16:refnum<k21>, "Error Out"=w18:errorcluster)  [unwired: 12 in]
  n113 = call <vilib>:"DMM Close.vi"("Instrument Handle In"=w16, "Error In"=w18) -> ("Error Out"=w26:errorcluster)  [unwired: 13 in]
  n114 = case shown="无错误" w26 {
    selector: w26 -> [_ w372]
    frame No Error {
      n115 = local write "测试进度"(u8 100 ("测试进度")) -> ()
    }
    frame Error {
      w373 = T6 3 items=["no dialog", "OK message", "continue or stop message", "OK message + warnings", "continue/stop + warnings"] ("type of dialog (OK msg:1)")
      n116 = call <vilib>:"Simple Error Handler.vi"("type of dialog (OK msg:1)"=w373, "error in (no error)"=w372) -> ()  [unwired: 3 in, 5 out]
    }
  }
